vi "Encrypt with AES-PORTABLE-5129.vi"(0 "Password.In":string, 2 "BitKeyType(256)":u16(ring)=256 items=["AES bit key 128"=128, "AES bit key 192"=192, "AES bit key 256"=256], 7 "Plain Text In":string, 11 "error in":errorcluster) -> (8 "Cyphered Text out":string, 15 "error out":errorcluster)   [LabVIEW 2020, in "Advanced Encryption Standard (AES).lvlib"]
doc: "Takes string (plain text) and encrypts it with Advanced Encryption Standart (AES) algorithm. \n\nThis VI allows reentrant execution."
uses:
  Advanced Encryption Standard (AES).lvlib
  Mix Bytes Phases Enum (Typedef).ctl
panel:
  out "cipherCharStr":string[](array[string])
  out "cipherChar":i32[](array[numeric])
  out "blockLength":i32
  out "cipherCntr":u16[](array[numeric])
  in  "0x100000000":u64=4294967296 format="%.0x"
  out "blockCount":i32
  in  "0xff":u16=255 format="%.0x"
  # "Number of bits used in the key (256 by default).\nThe longer a key, the higher level of protection\nat expence of processor and RAM usage."
  # "Advanced Encryption Standart (AES)\nAES Encrypt 1.0"
  # "Receives Password in String format (plain text)"
  # "Receives plain text needed to be encrypted"
  # "Encrypted text (with AES)"
  # "Development and Debugging"
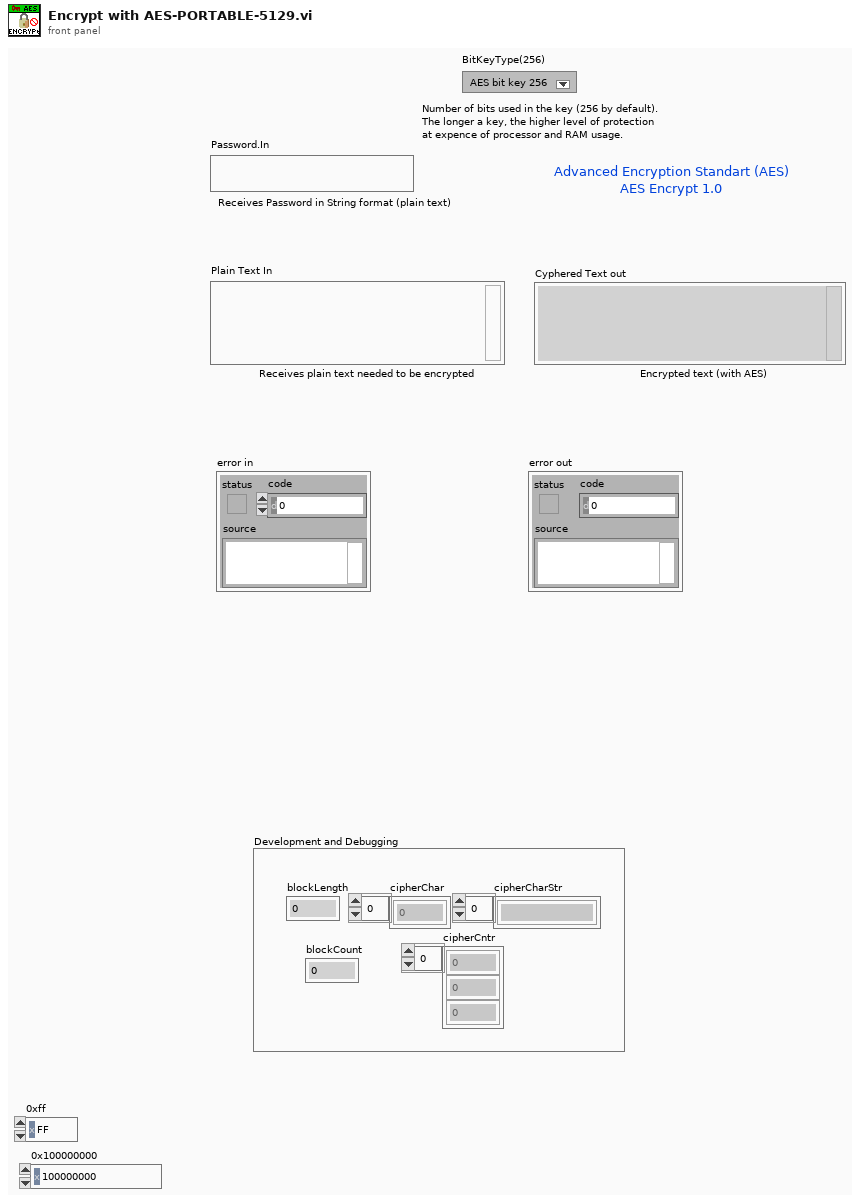
[diagram p1: front panel]
types:
  T1 = enum16{"Init", "Write pwBytes", "Create Key", "MixBlocks", "ToB64"}
  T2 = typedef "Mix Bytes Phases Enum (Typedef).ctl" = enum16{"Replace Blocks", "Cipher Blocks", "Replace ciphered", "Combine parts"}
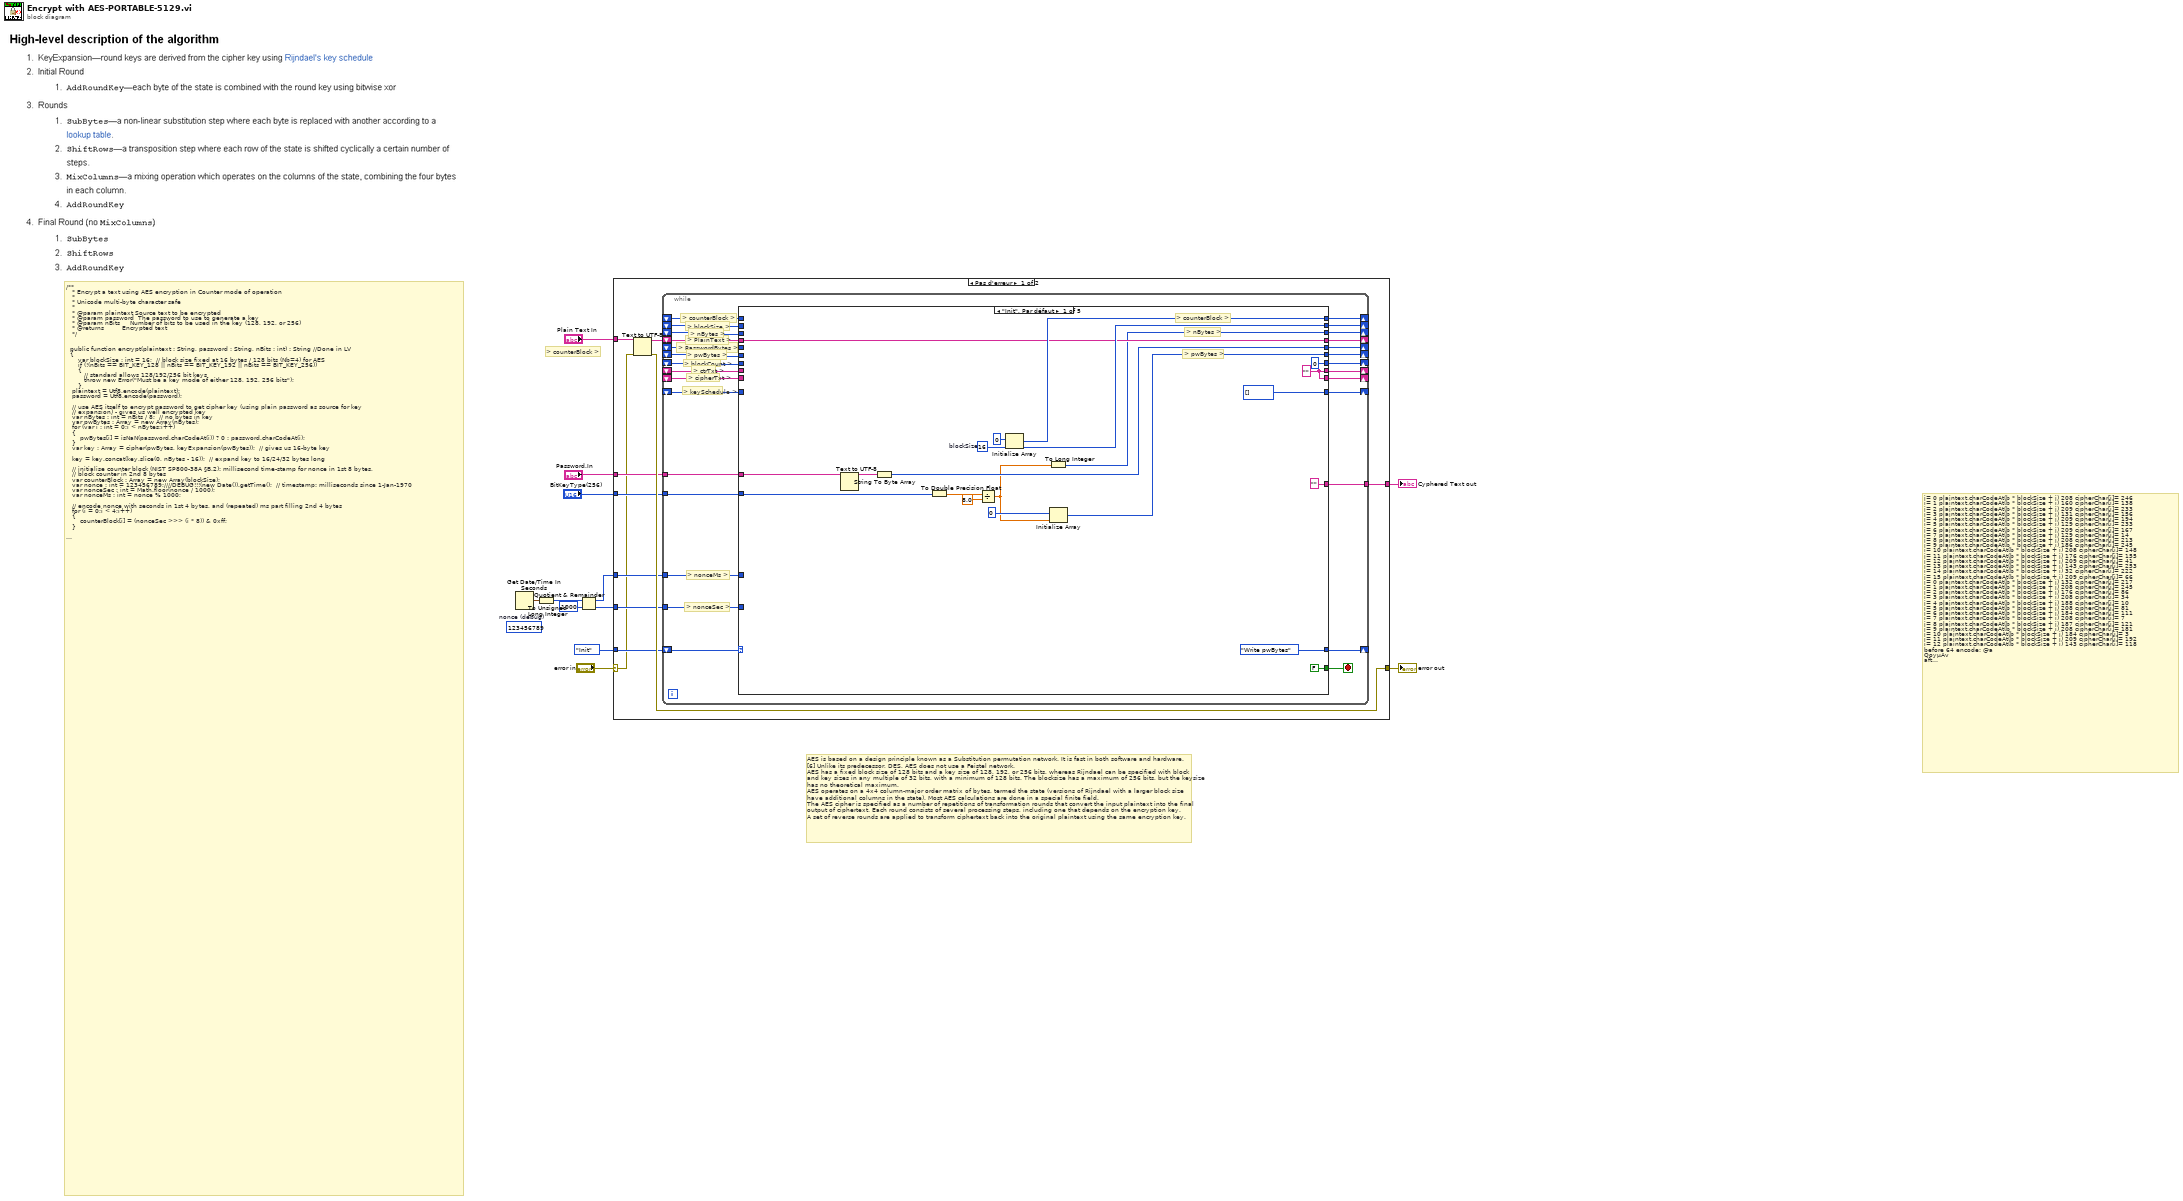
[diagram p0: block diagram]
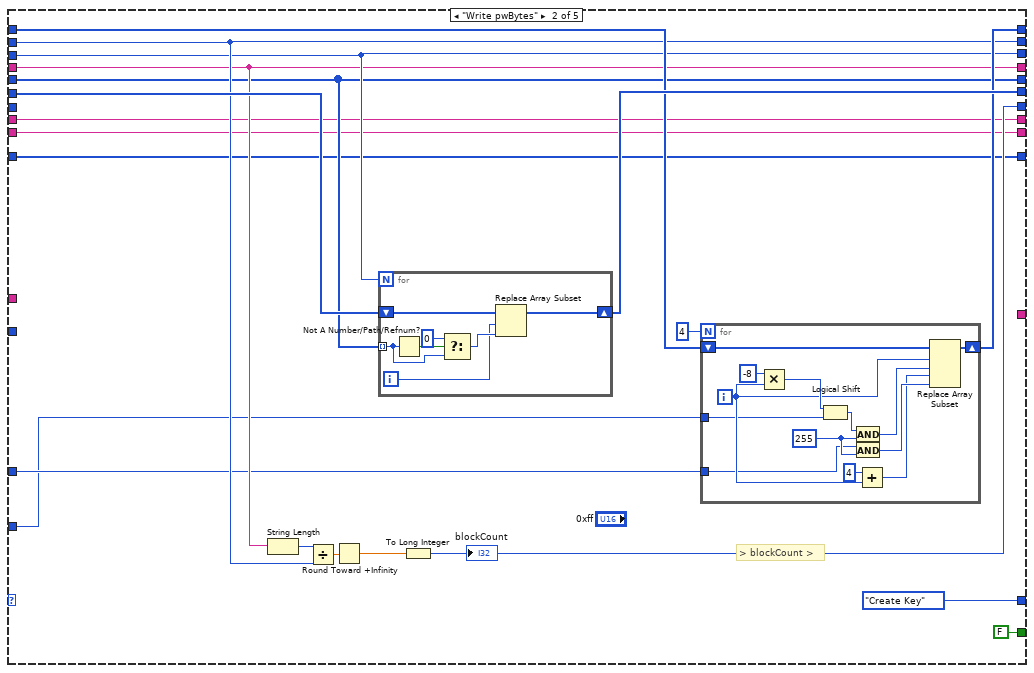
[diagram p2: hidden frame]
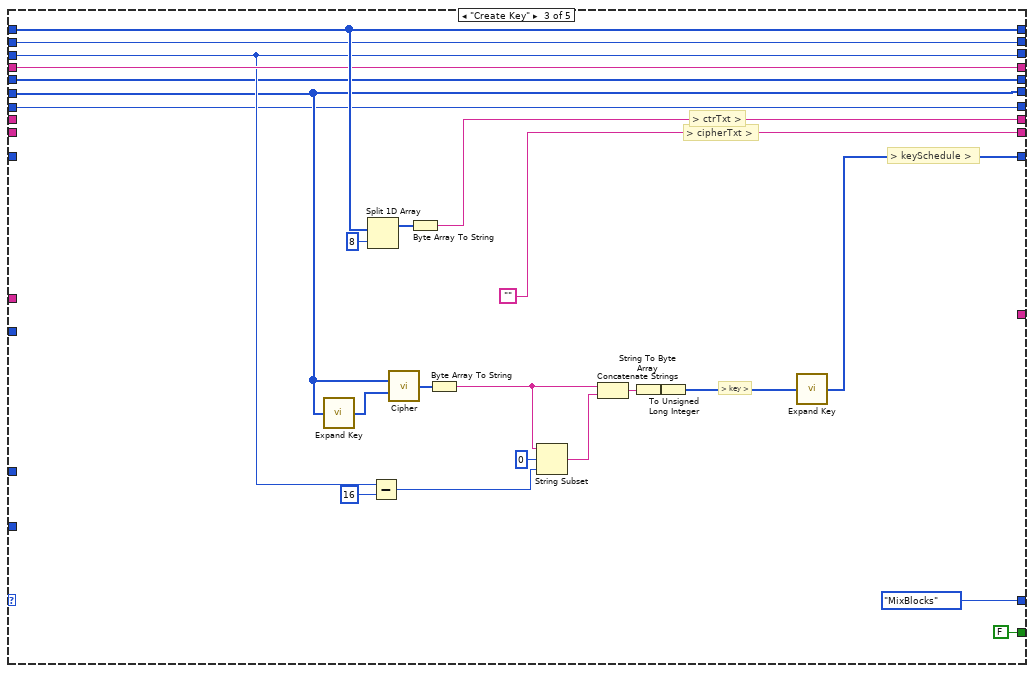
[diagram p3: hidden frame]
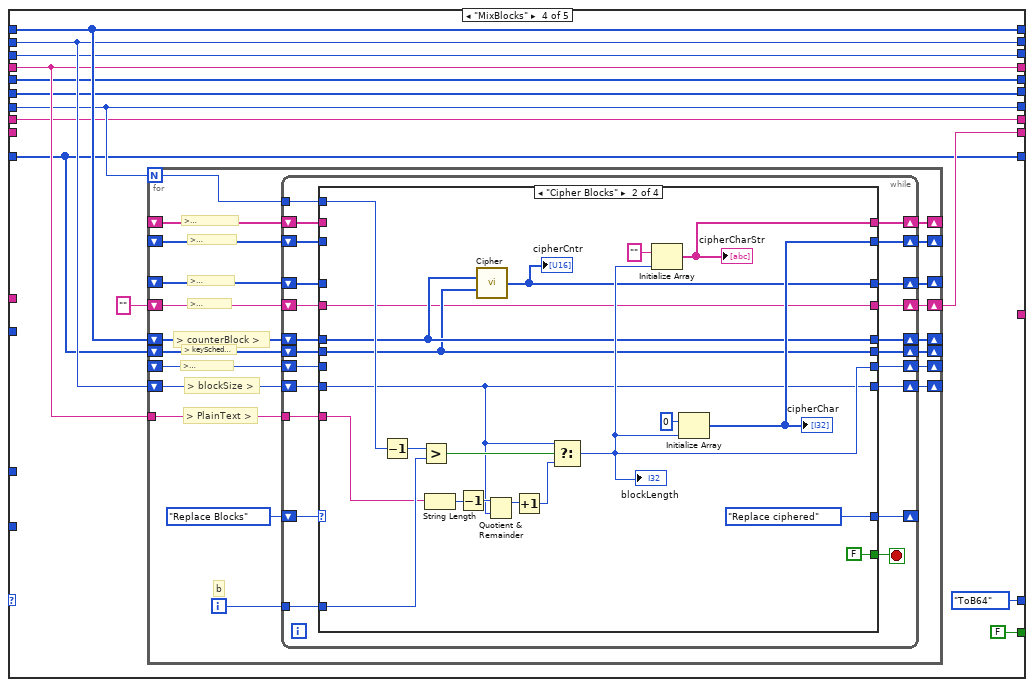
[diagram p4: hidden frame]
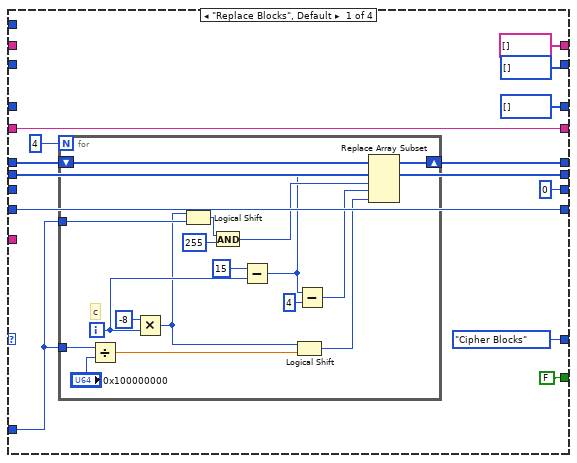
[diagram p5: hidden frame]
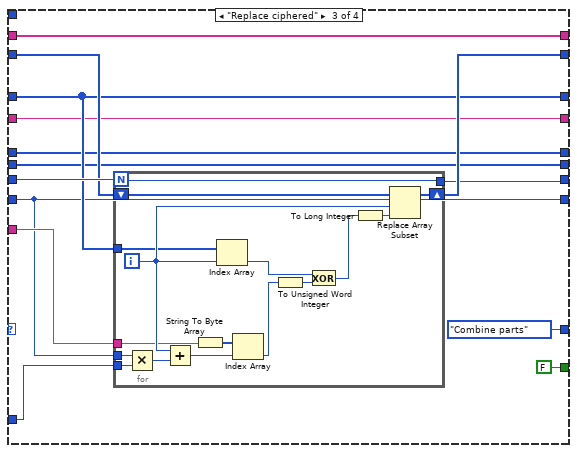
[diagram p6: hidden frame]
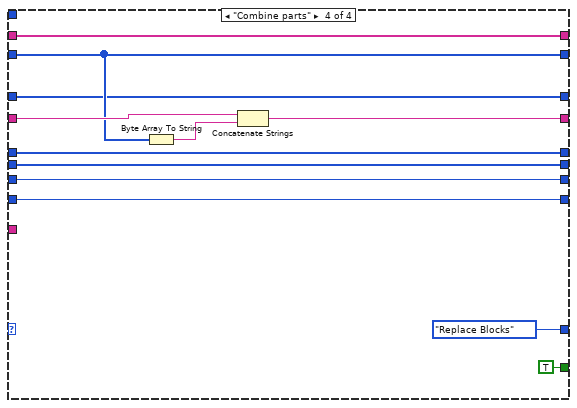
[diagram p7: hidden frame]
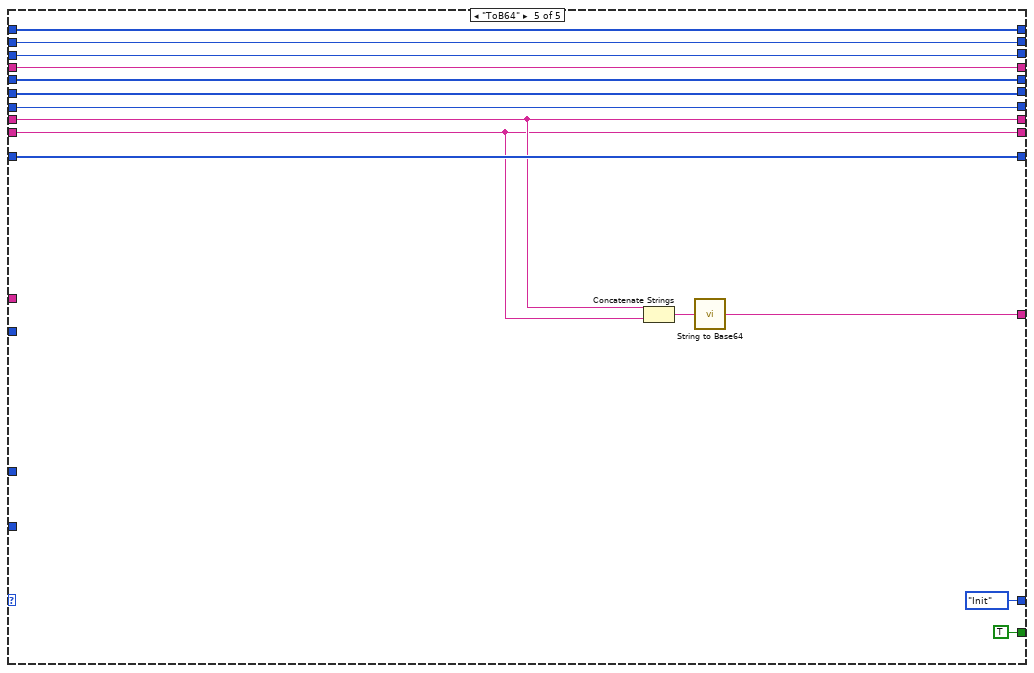
[diagram p8: hidden frame]
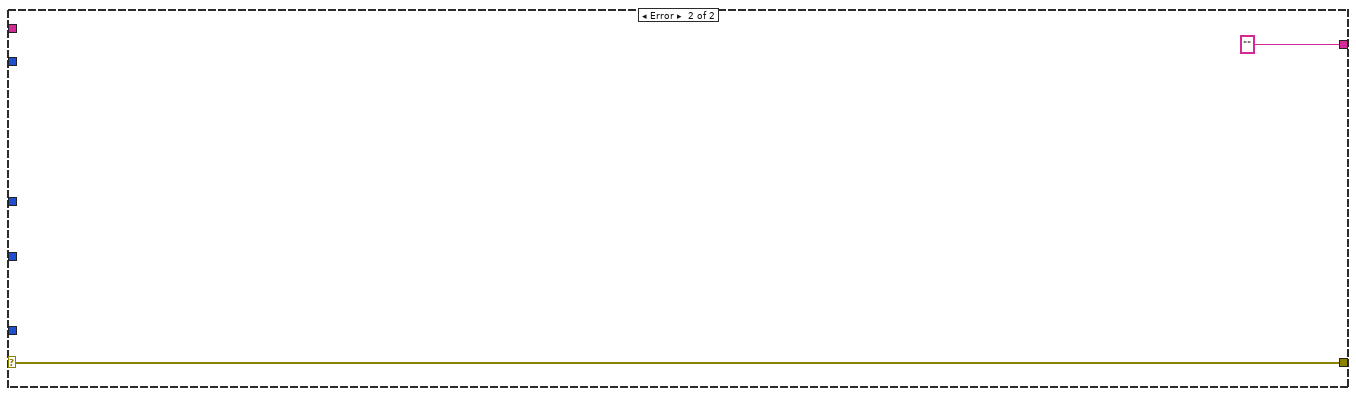
[diagram p9: hidden frame]
diagram:
  (unwired) u32 123456789  # nonce (debug)
  # "> counterBlock >"
  # "AES is based on a design principle known as a Substitution permutation network. It is fast in both software and hardware.\n[6] Unlike its predecessor, DES, AES does not use a Feistel network.\nAES has a fixed block size of 128 bits and a key size of 128, 192, or 256 bits, whereas Rijndael can be specified with block \nand key sizes in any multiple of 32 bits, with a minimum of 128 bits. The blocksize has a maximum of 256 bits, but the keysize \nhas no theoretical maximum.\nAES operates on a 4x4 column-major order matrix of bytes, termed the state (versions of Rijndael with a larger block size \nhave additional columns in the state). Most AES calculations are done in a special finite field.\nThe AES cipher is specified as a number of repetitions of transformation rounds that convert the input plaintext into the final \noutput of ciphertext. Each round consists of several processing steps, including one that depends on the encryption key. \nA set of reverse rounds are applied to transform ciphertext back into the original plaintext using the same encryption key."
  # "/** \n\t\t * Encrypt a text using AES encryption in Counter mode of operation\n\t\t *\n\t\t * Unicode multi-byte character safe\n\t\t *\n\t\t * @param plaintext Source text to be encrypted\n\t\t * @param password  The password to use to generate a key\n\t\t * @param nBits     Number of bits to be used in the key (128, 192, or 256)\n\t\t * @returns         Encrypted text\n\t\t */\n\t\t \n\t\t \n\t\tpublic function encrypt(plaintext : String, password : String, nBits : int) : String //Done in LV\n\t\t{\n\t\t\t   var blockSize : int = 16;  // block size fixed at 16 bytes / 128 bits (Nb=4) for AES\n\t\t   \tif (!(nBits == BIT_KEY_128 || nBits == BIT_KEY_192 || nBits == BIT_KEY_256)) \n      {\n\t\t\t\t     // standard allows 128/192/256 bit keys\n\t\t\t      throw new Error(\"Must be a key mode of either 128, 192, 256 bits\");\n\t\t   \t}\n\t\t\tplaintext = Utf8.encode(plaintext);\n\t\t\tpassword = Utf8.encode(password);\n\n\t\t\t// use AES itself to encrypt password to get cipher key (using plain password as source for key \n\t\t\t// expansion) - gives us well encrypted key\n\t\t\tvar nBytes : int = nBits / 8;  // no bytes in key\n\t\t\tvar pwBytes : Array = new Array(nBytes);\n\t\t\tfor (var i : int = 0;i < nBytes;i++) \n\t\t\t{\n\t\t\t\t   pwBytes[i] = isNaN(password.charCodeAt(i)) ? 0 : password.charCodeAt(i);\n\t\t\t}\n\t\t\tvar key : Array = cipher(pwBytes, keyExpansion(pwBytes));  // gives us 16-byte key\n\t\t\t\n\t\t\tkey = key.concat(key.slice(0, nBytes - 16));  // expand key to 16/24/32 bytes long\n\t\t\t\n\t\t\t// initialise counter block (NIST SP800-38A §B.2): millisecond time-stamp for nonce in 1st 8 bytes,\n\t\t\t// block counter in 2nd 8 bytes\n\t\t\tvar counterBlock : Array = new Array(blockSize);\n\t\t\tvar nonce : int = 123456789;////DEBUG!!!(new Date()).getTime();  // timestamp: milliseconds since 1-Jan-1970\n\t\t\tvar nonceSec : int = Math.floor(nonce / 1000);\n\t\t\tvar nonceMs : int = nonce % 1000;\n\t\t\t\n\t\t\t// encode nonce with seconds in 1st 4 bytes, and (repeated) ms part filling 2nd 4 bytes\n\t\t\tfor (i = 0;i < 4;i++) \n\t\t\t{\n\t\t\t\t   counterBlock[i] = (nonceSec >>> (i * 8)) & 0xff;\t\t\t\t\n\t\t\t}\n\t\t\t\n\t\t\tfor (i = 0;i < 4;i++)\n\t\t\t{\n\t\t\t\t   counterBlock[i + 4] = nonceMs & 0xff;\n\t\t\t} \n\t\t\t// and convert it to a string to go on the front of the ciphertext\n\t\t\tvar ctrTxt : String = '';\n\t\t\tfor (i = 0;i < 8;i++) \n\t\t\t{\n\t\t\t\t   ctrTxt += String.fromCharCode(counterBlock[i]);\n\t\t\t}\n\t\t\t// generate key schedule - an expansion of the key into distinct Key Rounds for each round\n\t\t\tvar keySchedule : Array = keyExpansion(key);\n\t\t\tvar blockCount : int = Math.ceil(plaintext.length / blockSize);\n\t\t\tvar ciphertxt : Array = new Array(blockCount);  // ciphertext as array of strings\n\t\t\t\n\t\t\tfor (var b : int = 0;b < blockCount;b++) \n\t\t\t{\n\t\t\t\t   // set counter (block #) in last 8 bytes of counter block (leaving nonce in 1st 8 bytes)\n\t\t\t\t   // done in two stages for 32-bit ops: using two words allows us to go past 2^32 blocks (68GB)\n\t\t\t\t   for (var c : int = 0;c < 4;c++) \n\t\t\t   \t{\n\t\t\t      \t\tcounterBlock[15 - c] = (b >>> (c * 8)) & 0xff;\t\t\t\t\t\n\t     \t}\n\t\t\t\t\n\t\t   \t\tfor (c = 0;c < 4;c++) \n\t\t   \t\t{\n\t\t      \t\t\tcounterBlock[15 - c - 4] = (b / 0x100000000 >>> c * 8);\n\t\t   \t\t}\n\t\t\t\t\n\t\t\t\tvar cipherCntr : Array = cipher(counterBlock, keySchedule);  // -- encrypt counter block --\n\t\t\t\t\n\t\t\t\t// block size is reduced on final block\n\t\t\t\tvar blockLength : int = b < blockCount - 1 ? blockSize : (plaintext.length - 1) % blockSize + 1;\n\t\t\t\tvar cipherChar : Array = new Array(blockLength);\n\t\t\t    \n\t\t\t\tfor (i = 0;i < blockLength;i++) \n\t\t\t\t{  \n\t\t\t   \t\t// -- xor plaintext with ciphered counter char-by-char --\n\t\t\t   \t\tcipherChar[i] = cipherCntr[i] ^ plaintext.charCodeAt(b * blockSize + i);\t\t\t\t\t\n\t\t   \t\t\t//trace(\"i=\",i,\"plaintext.charCodeAt(b * blockSize + i)\",plaintext.charCodeAt(b * blockSize + i),\"cipherChar[i]=\",cipherChar[i]);\n\t\t\t   \t\tcipherChar[i] = String.fromCharCode(cipherChar[i]);\n\t\t\t\t\t\n\t\t\t\t}\n\t\t\t\t\n\t\t\t\tciphertxt[b] = cipherChar.join(''); \n\t\t\t\t//trace(ciphertxt);\n\t\t\t}\n\t\t\t\n\t\t   \t// Array.join is more efficient than repeated string concatenation in IE\n\t\t   \tvar ciphertext : String = ctrTxt + ciphertxt.join('');\n\t   \t\t//trace(\"before 64 encode:\",ciphertext);\n   \t\t\tciphertext = Base64.encode(ciphertext);  // encode in base64\n\t\t\t   //trace(\"after 64 encode:\",ciphertext);\n\t\t\t   //alert((new Date()) - t);\n\t\t\t\n\t\t\treturn ciphertext;\n\t\t}"
  # "i= 0 plaintext.charCodeAt(b * blockSize + i) 208 cipherChar[i]= 246\ni= 1 plaintext.charCodeAt(b * blockSize + i) 160 cipherChar[i]= 138\ni= 2 plaintext.charCodeAt(b * blockSize + i) 209 cipherChar[i]= 233\ni= 3 plaintext.charCodeAt(b * blockSize + i) 131 cipherChar[i]= 156\ni= 4 plaintext.charCodeAt(b * blockSize + i) 209 cipherChar[i]= 194\ni= 5 plaintext.charCodeAt(b * blockSize + i) 129 cipherChar[i]= 233\ni= 6 plaintext.charCodeAt(b * blockSize + i) 209 cipherChar[i]= 167\ni= 7 plaintext.charCodeAt(b * blockSize + i) 129 cipherChar[i]= 14\ni= 8 plaintext.charCodeAt(b * blockSize + i) 208 cipherChar[i]= 213\ni= 9 plaintext.charCodeAt(b * blockSize + i) 186 cipherChar[i]= 245\ni= 10 plaintext.charCodeAt(b * blockSize + i) 208 cipherChar[i]= 148\ni= 11 plaintext.charCodeAt(b * blockSize + i) 176 cipherChar[i]= 155\ni= 12 plaintext.charCodeAt(b * blockSize + i) 209 cipherChar[i]= 41\ni= 13 plaintext.charCodeAt(b * blockSize + i) 143 cipherChar[i]= 253\ni= 14 plaintext.charCodeAt(b * blockSize + i) 32 cipherChar[i]= 222\ni= 15 plaintext.charCodeAt(b * blockSize + i) 209 cipherChar[i]= 66\ni= 0 plaintext.charCodeAt(b * blockSize + i) 132 cipherChar[i]= 217\ni= 1 plaintext.charCodeAt(b * blockSize + i) 208 cipherChar[i]= 245\ni= 2 plaintext.charCodeAt(b * blockSize + i) 176 cipherChar[i]= 86\ni= 3 plaintext.charCodeAt(b * blockSize + i) 208 cipherChar[i]= 34\ni= 4 plaintext.charCodeAt(b * blockSize + i) 188 cipherChar[i]= 10\ni= 5 plaintext.charCodeAt(b * blockSize + i) 208 cipherChar[i]= 81\ni= 6 plaintext.charCodeAt(b * blockSize + i) 184 cipherChar[i]= 111\ni= 7 plaintext.charCodeAt(b * blockSize + i) 208 cipherChar[i]= 7\ni= 8 plaintext.charCodeAt(b * blockSize + i) 187 cipherChar[i]= 121\ni= 9 plaintext.charCodeAt(b * blockSize + i) 208 cipherChar[i]= 181\ni= 10 plaintext.charCodeAt(b * blockSize + i) 184 cipherChar[i]= 3\ni= 11 plaintext.charCodeAt(b * blockSize + i) 209 cipherChar[i]= 192\ni= 12 plaintext.charCodeAt(b * blockSize + i) 143 cipherChar[i]= 118\nbefore 64 encode: @a\nQoyµAv\nafter 64 encode: QOIBABUVFRX2iumcwumnDtX1lJsp/d5C2fVWIgpRbwd5tQPAdj=="
  n1 = Get Date/Time In Seconds() -> (seconds since 1Jan1904=w2:timestamp)
  n2 = To Unsigned Long Integer(number=w2) -> (unsigned 32bit integer=w1:u32)
  n3 = Quotient & Remainder(x=w1, y=u32 1000) -> (x-y*floor(x/y)=w9:u32, floor(x/y)=w8:u32)
  n4 = case shown="Pas d'erreur" "error in" {
    selector: "error in" -> [w13 w298]
    tunnel: [w21 w298] -> w11
    tunnel: T1."Init" ("Encryption Phases") -> [w20 _]
    tunnel: w9 -> [w19 _]
    tunnel: w8 -> [w18 _]
    tunnel: "Plain Text In" -> [w17 _]
    tunnel: "Password.In" -> [w16 _]
    tunnel: "BitKeyType(256)" -> [w15 _]
    tunnel: [w14 "" ("Base64 String")] -> w4
    frame No Error {
      n5 = Text to UTF-8(8:w13, 11:w17) -> (0:w21:errorcluster, 3:w22:string)  [unwired: 1 in]
      n6 = while {
        shift-right: [w34] -> _
        shift-left: w20 -> [w50]
        tunnel: w16 -> [w49]
        tunnel: w15 -> [w48]
        shift-right: [w46] -> _
        shift-left: _ -> [w42]
        shift-right: [w45] -> _
        shift-left: _ -> [w41]
        shift-right: [w44] -> _
        shift-left: _ -> [w43]
        shift-right: [w33] -> _
        shift-left: w22 -> [w47]
        shift-right: [w40] -> _
        shift-left: _ -> [w39]
        shift-right: [w38] -> _
        shift-left: _ -> [w37]
        shift-right: [w36] -> _
        shift-left: _ -> [w35]
        shift-right: [w32] -> _
        shift-left: _ -> [w31]
        shift-right: [w30] -> _
        shift-left: _ -> [w29]
        shift-right: [w28] -> _
        shift-left: _ -> [w27]
        tunnel: [w25] -> w14
        tunnel: w19 -> [w24]
        tunnel: w18 -> [w23]
        stop <- w26 stop-if-true
        # "> nonceSec >"
        # "> nonceMs >"
        # "> keySchedule >"
        # "> cipherTxt >"
        # "> ctrTxt >"
        # "> PasswordBytes >"
        # "> blockCount >"
        # "> blockSize >"
        # "> counterBlock >"
        # "> nBytes >"
        # "> PlainText >"
        # "> pwBytes >"
        n7 = case shown="\"Init\", Par défaut" w50 {
          tunnel: w49 -> [w67 _ _ _ _]
          tunnel: w48 -> [w53 _ _ _ _]
          tunnel: w47 -> [w61 w79 w119 w143 w290]
          tunnel: [w55 w80 w118 w144 w291] -> w46
          tunnel: [w66 w78 w117 w142 w289] -> w45
          tunnel: [w65 w86 w116 w141 w288] -> w44
          tunnel: w43 -> [_ w87 w116 w141 w288]
          tunnel: w42 -> [_ w80 w118 w144 w291]
          tunnel: w41 -> [_ w78 w117 w142 w289]
          tunnel: [w64 w84 w124 w146 w293] -> w40
          tunnel: w39 -> [_ w85 w124 w146 w293]
          tunnel: [w63 w83 w120 w145 w292] -> w38
          tunnel: w37 -> [_ w83 w120 w145 w292]
          tunnel: [0 w81 w115 w140 w287] -> w36
          tunnel: w35 -> [_ _ w115 w140 w287]
          tunnel: [T1."Write pwBytes" ("Encryption Phases") T1."Create Key" ("Encryption Phases") T1."MixBlocks" ("Encryption Phases") T1."ToB64" ("Encryption Phases") T1."Init" ("Encryption Phases")] -> w34
          tunnel: [w61 w79 w119 w143 w290] -> w33
          tunnel: [w60 w77 w123 w139 w285] -> w32
          tunnel: w31 -> [_ w77 _ w139 w285]
          tunnel: [w60 w76 "" w147 w284] -> w30
          tunnel: w29 -> [_ w76 _ _ w284]
          tunnel: [u16[] [] ("ExpandedKey") w75 w121 w138 w286] -> w28
          tunnel: w27 -> [_ w75 _ w138 w286]
          tunnel: [FALSE FALSE FALSE FALSE TRUE] -> w26
          tunnel: ["" ("Base64 String") _ _ _ w294] -> w25
          tunnel: w24 -> [_ w74 _ _ _]
          tunnel: w23 -> [_ w73 _ _ _]
          frame "Init", Default {
            w63 = 16  # blockSize
            w60 = "" ("string")
            # "> counterBlock >"
            # "> pwBytes >"
            # "> nBytes >"
            n8 = Text to UTF-8(11:w67) -> (3:w70:string)  [unwired: 2 in, 1 out]
            n9 = String To Byte Array(string=w70) -> (unsigned byte array=w66:u8[])
            n10 = To Double Precision Float(number=w53) -> (double precision float=w52:dbl)
            n11 = Divide(x=w52, y=8.0) -> (x/y=w62:dbl)
            n12 = Initialize Array(u32 0 ("y"), w63) -> (w64:u32[])
            n13 = To Long Integer(number=w62) -> (32bit integer=w55:i32)
            n14 = Initialize Array(u32 0 ("element"), w62) -> (w65:u32[])
          }
          frame "Write pwBytes" {
            # "> blockCount >"
            n15 = String Length(string=w79) -> (length=w89:i32)
            n16 = Divide(x=w89, y=w83) -> (x/y=w90:dbl)
            n17 = Round Toward +Infinity(x=w90) -> (ceil(x): smallest int >= x=w82:dbl)
            n18 = for {
              N: w80 -> [_]
              tunnel: w78 -> [w106] mode=indexing
              shift-right: [w105] -> w86
              shift-left: w87 -> [w104]
              i -> [w108]
              n19 = Not A Number/Path/Refnum?(number/path/refnum=w106) -> (NaN/Path/Refnum?=w110:bool)
              n20 = Select(t=0 ("f"), s=w110, f=w106) -> (s? t:f=w109:i32)
              n21 = Replace Array Subset(array=w104, new element=w109, index=w108) -> (w105:u32[])
            }
            n22 = To Long Integer(number=w82) -> (32bit integer=w81:i32)
            "blockCount" <- w81
            n23 = for {
              N: 4 -> [_]
              shift-right: [w95] -> w84
              shift-left: w85 -> [w94]
              tunnel: w74 -> [w92]
              tunnel: w73 -> [w91]
              i -> [w98]
              w93 = u16 255 ("0xff")
              n24 = Multiply(x=-8, y=w98) -> (x*y=w102:i32)
              n25 = Logical Shift(y=w102, x=w91) -> (x << y=w101:u32)
              n26 = And(x=w101, y=w93) -> (x .and. y?=w100:u32)
              n27 = And(x=w92, y=w93) -> (x .and. y?=w97:u32)
              n28 = Add(x=4, y=w98) -> (x+y=w96:i32)
              n29 = Replace Array Subset(array=w94, new element #1=w100, index #1=w98, new element #2=w97, index #2=w96) -> (w95:u32[])
            }
          }
          frame "Create Key" {
            # "> keySchedule >"
            # "> cipherTxt >"
            # "> ctrTxt >"
            # "> key >"
            n30 = call "Expand Key.vi"("Key"=w116) -> ("Expanded Key"=w125:u32[])  [unwired: 13 in, 1 out]
            n31 = Split 1D Array(array=w124, index=8) -> (first subarray=w134:u32[])  [unwired: 1 out]
            n32 = Subtract(x=w118, y=u8 16) -> (x-y=w130:i32)
            n33 = call "Cipher.vi"("Key(input)"=w116, "ExpandedKey(w)1D"=w125) -> ("Cypher Output"=w126:u16[])  [unwired: 12 in, 1 out]
            n34 = Byte Array To String(unsigned byte array=w134) -> (string=w123:string)
            n35 = Byte Array To String(unsigned byte array=w126) -> (string=w127:string)
            n36 = String Subset(string=w127, offset (0)=0, length (rest)=w130) -> (substring=w131:string)
            n37 = Concatenate Strings(w127, w131) -> (w132:string)
            n38 = String To Byte Array(string=w132) -> (unsigned byte array=w114:u8[])
            n39 = To Unsigned Long Integer(number=w114) -> (unsigned 32bit integer=w113:u32[])
            n40 = call "Expand Key.vi"("Key"=w113) -> ("Expanded Key"=w121:u32[])  [unwired: 13 in, 1 out]
          }
          frame "MixBlocks" {
            n41 = for {
              N: w140 -> [w163]
              shift-right: [w165] -> _
              shift-left: w146 -> [w166]
              shift-right: [w149] -> _
              shift-left: w138 -> [w164]
              shift-right: [w154] -> _
              shift-left: w145 -> [w162]
              tunnel: w143 -> [w161]
              shift-right: [w160] -> _
              shift-left: _ -> [w159]
              shift-right: [w158] -> _
              shift-left: _ -> [w157]
              shift-right: [w156] -> _
              shift-left: _ -> [w155]
              shift-right: [w153] -> _
              shift-left: _ -> [w152]
              shift-right: [w151] -> w147
              shift-left: "" -> [w150]
              i -> [w167]
              # "> cipherTxt >"
              # "> cipherCntr >"
              # "> blockLength >"
              # "> cipherChar >"
              # "> cipherCharStr >"
              # "> PlainText >"
              # "> blockSize >"
              # "> keySchedule >"
              # "> counterBlock >"
              # "b"
              n42 = while {
                shift-right: [w188] -> _
                shift-left: Mix_Bytes_Phases_Enum_(Typedef)."Replace Blocks" ("Mix Bytes Phases") -> [w189]
                tunnel: w167 -> [w186]
                shift-right: [w184] -> w165
                shift-left: w166 -> [w185]
                shift-right: [w181] -> w149
                shift-left: w164 -> [w183]
                tunnel: w163 -> [w182]
                shift-right: [w168] -> w154
                shift-left: w162 -> [w180]
                tunnel: w161 -> [w179]
                shift-right: [w178] -> w160
                shift-left: w159 -> [w169]
                shift-right: [w177] -> w158
                shift-left: w157 -> [w174]
                shift-right: [w176] -> w156
                shift-left: w155 -> [w175]
                shift-right: [w173] -> w153
                shift-left: w152 -> [w172]
                shift-right: [w171] -> w151
                shift-left: w150 -> [w170]
                stop <- w187 stop-if-true
                n43 = case shown="\"Cipher Blocks\"" w189 {
                  tunnel: [Mix_Bytes_Phases_Enum_(Typedef)."Cipher Blocks" ("Mix Bytes Phases") Mix_Bytes_Phases_Enum_(Typedef)."Replace ciphered" ("Mix Bytes Phases") Mix_Bytes_Phases_Enum_(Typedef)."Combine parts" ("Mix Bytes Phases") Mix_Bytes_Phases_Enum_(Typedef)."Replace Blocks" ("Mix Bytes Phases")] -> w188
                  tunnel: [FALSE FALSE FALSE TRUE] -> w187
                  tunnel: w186 -> [w200 w232 w254 _]
                  tunnel: w185 -> [w199 w225 w245 w275]
                  tunnel: [w198 w225 w245 w275] -> w184
                  tunnel: w183 -> [w197 w224 w244 w274]
                  tunnel: w182 -> [_ w231 _ _]
                  tunnel: [w197 w224 w244 w274] -> w181
                  tunnel: w180 -> [w193 w223 w246 w273]
                  tunnel: w179 -> [_ w230 w251 _]
                  tunnel: [string[] [] w229 w249 w278] -> w178
                  tunnel: [i32[] [] w228 w250 w277] -> w177
                  tunnel: [0 ("blockSize") w227 w247 w272] -> w176
                  tunnel: w175 -> [_ _ w253 w272]
                  tunnel: w174 -> [_ _ w252 w277]
                  tunnel: [u16[] [] ("Cypher.Output") w226 w248 w276] -> w173
                  tunnel: w172 -> [_ _ w248 w276]
                  tunnel: [w191 w222 w243 w280] -> w171
                  tunnel: w170 -> [w191 w222 w243 w279]
                  tunnel: w169 -> [_ _ w249 w278]
                  tunnel: [w193 w223 w246 w273] -> w168
                  frame "Replace Blocks", Default {
                    n44 = for {
                      N: 4 -> [_]
                      tunnel: w200 -> [w217]
                      tunnel: w200 -> [w210]
                      shift-right: [w203] -> w198
                      shift-left: w199 -> [w204]
                      i -> [w216]
                      # "c"
                      n45 = Divide(x=w210, y="0x100000000") -> (x/y=w208:dbl)
                      n46 = Multiply(x=-8, y=w216) -> (x*y=w209:i32)
                      n47 = Logical Shift(y=w209, x=w217) -> (x << y=w219:i32)
                      n48 = And(x=w219, y=u16 255 ("0xff")) -> (x .and. y?=w214:i32)
                      n49 = Subtract(x=15, y=w216) -> (x-y=w213:i32)
                      n50 = Logical Shift(y=w209, x=w208) -> (x << y=w207:u32)
                      n51 = Subtract(x=w213, y=4) -> (x-y=w211:i32)
                      n52 = Replace Array Subset(array=w204, new element #1=w214, index #1=w213, new element #2=w207, index #2=w211) -> (w203:u32[])
                    }
                  }
                  frame "Cipher Blocks" {
                    n53 = Decrement(x=w231) -> (x-1=w233:i32)
                    n54 = Greater?(x=w233, y=w232) -> (0:w234:bool)
                    n55 = String Length(string=w230) -> (length=w236:i32)
                    n56 = Decrement(x=w236) -> (x-1=w235:i32)
                    n57 = call "Cipher.vi"("Key(input)"=w225, "ExpandedKey(w)1D"=w224) -> ("Cypher Output"=w226:u16[])  [unwired: 12 in, 1 out]
                    "cipherCntr" <- w226
                    n58 = Quotient & Remainder(x=w235, y=w223) -> (x-y*floor(x/y)=w237:i32)  [unwired: 1 out]
                    n59 = Increment(x=w237) -> (x+1=w238:i32)
                    n60 = Select(t=w223, s=w234, f=w238) -> (s? t:f=w227:i32)
                    "blockLength" <- w227
                    n61 = Initialize Array("", w227) -> (w229:string[])
                    "cipherCharStr" <- w229
                    n62 = Initialize Array(0, w227) -> (w228:i32[])
                    "cipherChar" <- w228
                  }
                  frame "Replace ciphered" {
                    n63 = for {
                      N: w253 -> [w259]
                      tunnel: w254 -> [w268]
                      shift-right: [w263] -> w250
                      shift-left: w252 -> [w264]
                      tunnel: w246 -> [w262]
                      tunnel: w251 -> [w261]
                      tunnel: w248 -> [w260]
                      tunnel: [w259] -> w247
                      i -> [w265]
                      n64 = Multiply(x=w262, y=w268) -> (x*y=w267:i32)
                      n65 = Add(x=w265, y=w267) -> (x+y=w266:i32)
                      n66 = String To Byte Array(string=w261) -> (unsigned byte array=w269:u8[])
                      n67 = Index Array(array=w260, index=w265) -> (element=w270:u16)
                      n68 = Index Array(array=w269, index=w266) -> (element=w257:u8)
                      n69 = To Unsigned Word Integer(number=w257) -> (unsigned 16bit integer=w258:u16)
                      n70 = Exclusive Or(1:w258, 2:w270) -> (0:w255:u16)
                      n71 = To Long Integer(number=w255) -> (32bit integer=w256:i32)
                      n72 = Replace Array Subset(array=w264, new element=w256, index=w265) -> (w263:i32[])
                    }
                  }
                  frame "Combine parts" {
                    n73 = Byte Array To String(unsigned byte array=w277) -> (string=w281:string)
                    n74 = Concatenate Strings(w279, w281) -> (w280:string)
                  }
                }
              }
            }
          }
          frame "ToB64" {
            n75 = Concatenate Strings(w285, w284) -> (w296:string)
            n76 = call "String to Base64.vi"("Plain String"=w296) -> ("Base64 String"=w294:string)  [unwired: 13 in, 1 out]
          }
        }
      }
    }
    frame Error {
    }
  }
  "error out" <- w11
  "Cyphered Text out" <- w4
